vi "站点信息设置.vi"() -> ()   [LabVIEW 2016]
uses:
  <vilib>/Utility/miscctls.llb/LVPointTypeDef.ctl
  <vilib>/Utility/config.llb/NI_LVConfig.lvlib
panel:
  in  "title":string
  in  "站点系列号":string
  in  "站点名称":string
  in  "布尔":bool
  in  "取消":bool
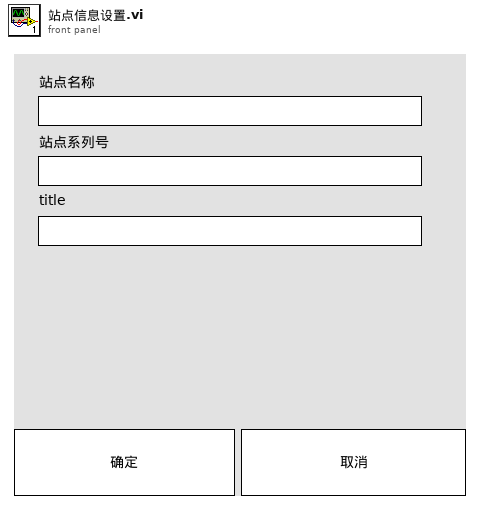
[diagram p1: front panel]
types:
  T1 = typedef "LVPointTypeDef.ctl" = cluster{"Horizontal":i16, "Vertical":i16}
  T2 = typedef "NI_LVConfig.lvlib/Config Data RefNum.ctl" = refnum<k1>
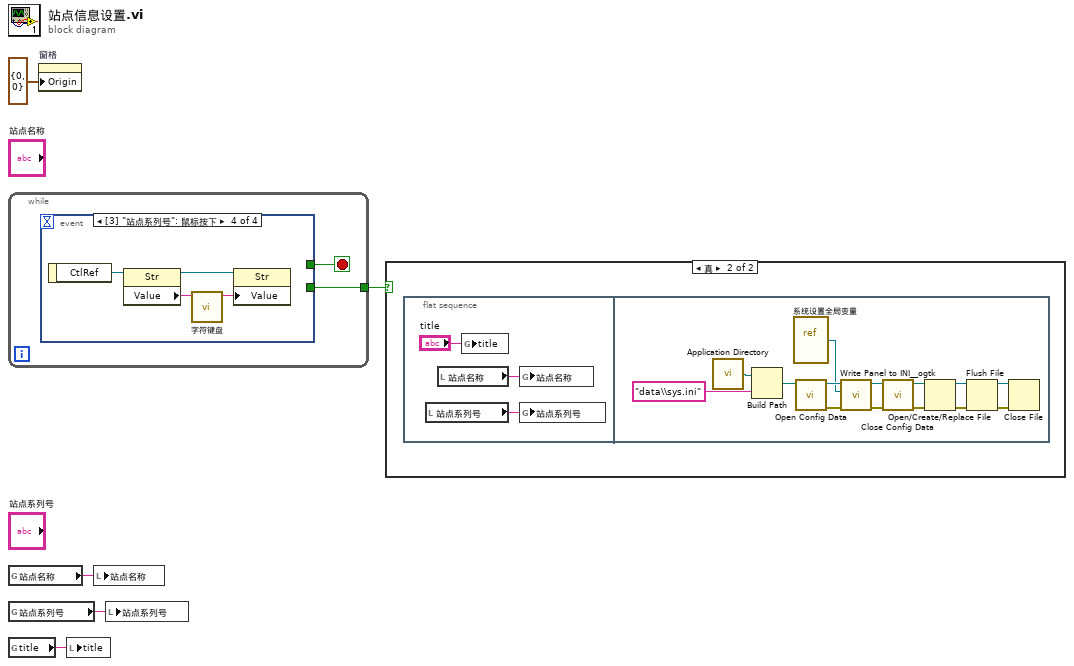
[diagram p0: block diagram]
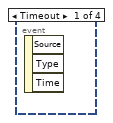
[diagram p3: hidden frame]
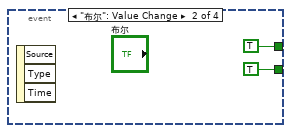
[diagram p4: hidden frame]
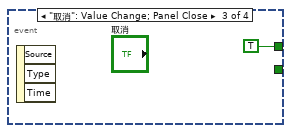
[diagram p5: hidden frame]
diagram:
  n1 = while {
    tunnel: [w6] -> w2
    stop <- w7 stop-if-true
    n2 = event shown="[3] \"站点系列号\": 鼠标按下" {
      selector: _ -> [_ _ _ _]
      dyn-events: _ -> [_ _ _ _]
      timeout: _ -> [_ _ _ _]
      tunnel: [_ TRUE TRUE _] -> w7
      tunnel: [_ TRUE _ _] -> w6
      event Timeout {
        n3 = event-data() -> ()  [unwired: 1 in, 3 out]
      }
      event "布尔": Value Change {
        n4 = event-data() -> ()  [unwired: 1 in, 3 out]
      }
      event "取消": Value Change; Panel Close {
        n5 = event-data() -> ()  [unwired: 1 in, 3 out]
      }
      event "站点系列号": Mouse Down {
        n6 = event-data() -> ("CtlRef"=w14:refnum<vi>)  [unwired: 1 in]
        n7 = property class="Str"(reference=w14) -> (reference out=w11:refnum<vi>, "Value"=w13:string)  [unwired: 1 in, 1 out]
        n8 = call "字符键盘.vi"("Old String"=w13) -> ("String"=w12:string)  [unwired: 10 in]
        n9 = property class="Str"(reference=w11, "Value"=w12) -> ()  [unwired: 1 in, 2 out]
      }
    }
  }
  n10 = global read "系统设置全局变量.vi" "站点名称"() -> (w4:string)
  n11 = global read "系统设置全局变量.vi" "站点系列号"() -> (w3:string)
  n12 = global read "系统设置全局变量.vi" "title"() -> (w1:string)
  n13 = property on="窗格" class="Pane"("Origin"=T1 {"Horizontal"=0, "Vertical"=0} ("原点")) -> ()  [unwired: 2 in, 2 out]
  n14 = local write "title"(w1) -> ()
  n15 = local write "站点名称"(w4) -> ()
  n16 = local write "站点系列号"(w3) -> ()
  n17 = case shown="真" w2 {
    frame False {
    }
    frame True {
      n18 = flat-sequence {
        frame #0 {
          n19 = local read "站点系列号"() -> (w17:string)
          n20 = local read "站点名称"() -> (w16:string)
          n21 = global write "系统设置全局变量.vi" "title"("title") -> ()
          n22 = global write "系统设置全局变量.vi" "站点名称"(w16) -> ()
          n23 = global write "系统设置全局变量.vi" "站点系列号"(w17) -> ()
        }
        frame #1 {
          n24 = call <vilib>:"Application Directory.vi"() -> ("Application Directory"=w31:path)
          n25 = Build Path(base path=w31, name or relative path="data\\sys.ini" ("名称或相对路径")) -> (appended path=w29:path)
          n26 = vi-ref "系统设置全局变量.vi"() -> (w27:refnum<vi>)
          n27 = call <vilib>:"Open Config Data.vi"("configuration file path"=w29) -> ("error out"=w25:errorcluster, "refnum"=w28:T2)  [unwired: 8 in, 1 out]
          n28 = call <userlib>:"Write Panel to INI__ogtk.vi"("error in (no error)"=w25, "VI ref"=w27, "refnum"=w28) -> ("error out"=w24:errorcluster, "refnum out"=w26:T2)  [unwired: 7 in]
          n29 = call <vilib>:"Close Config Data.vi"("error in (no error)"=w24, "refnum"=w26) -> ("error out"=w19:errorcluster, "file path"=w18:path)  [unwired: 8 in]
          n30 = Open/Create/Replace File(file path (use dialog)=w18, error in=w19) -> (refnum out=w22:refnum<file>, error out=w23:errorcluster)  [unwired: 4 in, 1 out]
          n31 = Flush File(refnum=w22, error in=w23) -> (refnum out=w21:refnum<file>, error out=w20:errorcluster)
          n32 = Close File(refnum=w21, error in=w20) -> ()  [unwired: 2 out]
        }
      }
    }
  }
